vi "LstCreateAndCombineDevice.vi"(8 "error in (no error)":errorcluster, 9 "dwCount in":u32, 10 "pDevicesHandles in":u32[](array[numeric])) -> (0 "error out":errorcluster, 1 "dwCount out":u32, 2 "pDevicesHandles out":u32[](array[numeric]), 3 "hDevice":u32)   [LabVIEW 2018, in "LibTiePie.lvlib"]
uses:
  LibTiePie.lvlib
  LabViewHS4/libtiepie.dll
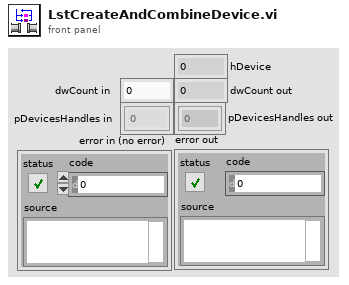
[diagram p1: front panel]
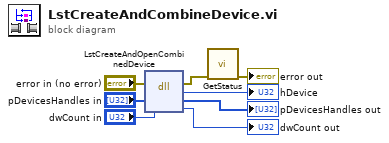
[diagram p0: block diagram]
diagram:
  n1 = dll-call lib="C:/Users/cwaha/Documents/LabViewHS4/libtiepie.dll" fn="LstCreateAndOpenCombinedDevice"(error in="error in (no error)", "pDevicesHandles"="pDevicesHandles in", "dwCount"="dwCount in") -> (error out=w4:errorcluster, "hDevice"=→"hDevice":u32, "pDevicesHandles"=→"pDevicesHandles out":u32[], "dwCount"=→"dwCount out":u32)  [unwired: 2 in, 1 out]
  n2 = call "GetStatus.vi"("error in (no error)"=w4) -> ("error out"=→"error out":errorcluster)  [unwired: 10 in]
